vi "CamDef.vi"() -> ()   [LabVIEW 2009]
panel:
  out "CamDef":bool
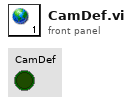
[diagram p1: front panel]
diagram:
